vi "Stepper FPGA Solution.vi"() -> ()   [LabVIEW 2012]
uses:
  <vilib>/rvi/eio/common/nirviEmuTemplateMethod_errors.vi
  <vilib>/eio/EIONode/EIONode.xnode
panel:
  in  "Step Period":i16
  in  "Direction":bool
  in  "Enable/Disable":bool
  out "Step Period":i16
  in  "Stop":bool
  out "Edge Count":i32
  out "Heartbeat":bool
  out "Absolute Position":i16
  # "Motor Feedback"
  # "Motor Command"
  # "Calibrate Steps to Deg"
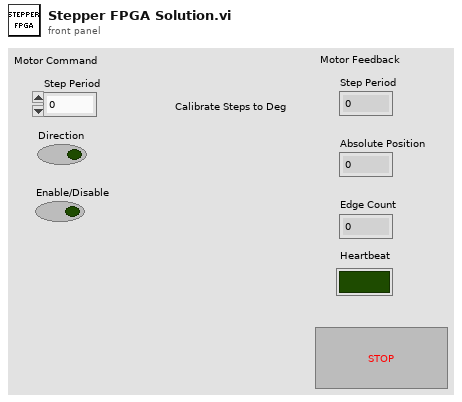
[diagram p1: front panel]
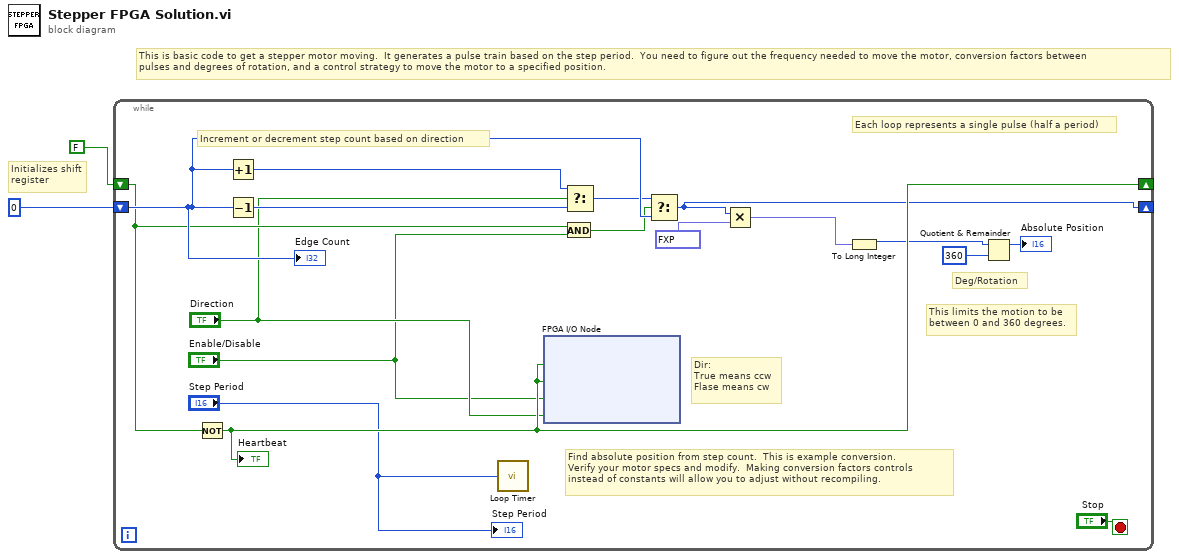
[diagram p0: block diagram]
diagram:
  # "Initializes shift\nregister"
  # "This is basic code to get a stepper motor moving.  It generates a pulse train based on the step period.  You need to figure out the frequency needed to move the motor, conversion factors between \npulses and degrees of rotation, and a control strategy to move the motor to a specified position."
  n1 = while {
    shift-right: [w9] -> _
    shift-left: i16 0 -> [w19]
    shift-right: [w16] -> _
    shift-left: FALSE -> [w17]
    stop <- "Stop" stop-if-true
    # "This limits the motion to be\nbetween 0 and 360 degrees."
    # "Deg/Rotation"
    # "Each loop represents a single pulse (half a period)"
    # "Dir:\nTrue means ccw\nFlase means cw"
    # "Find absolute position from step count.  This is example conversion.  \nVerify your motor specs and modify.  Making conversion factors controls\ninstead of constants will allow you to adjust without recompiling."
    # "Increment or decrement step count based on direction"
    n2 = Not(x=w17) -> (.not. x?=w16:bool)
    "Heartbeat" <- w16
    n3 = Increment(x=w19) -> (x+1=w15:i16)
    n4 = Decrement(x=w19) -> (x-1=w14:i16)
    n5 = call "Loop Timer"("Count(Ticks)"="Step Period") -> ()  [unwired: 1 out]
    n6 = xnode "FPGA I/O Node"("Stepper_Step"=w16, "Heartbeat LED"=w16, "Stepper_Enable"="Enable/Disable", "Stepper_Direction"="Direction") -> ()  [unwired: 4 in, 4 out]
    n7 = And(x=w17, y="Enable/Disable") -> (x .and. y?=w11:bool)
    n8 = Select(t=w15, s="Direction", f=w14) -> (s? t:f=w13:i16)
    n9 = Select(t=w13, s=w11, f=w19) -> (s? t:f=w9:i16)
    n10 = Multiply(x=w9, y=fxp<+,5,0> 0.90625) -> (x*y=w4:fxp<+/-,21,16>)
    n11 = To Long Integer(number=w4) -> (32bit integer=w3:i32)
    n12 = Quotient & Remainder(x=w3, y=i16 360) -> (x-y*floor(x/y)=→"Absolute Position":i32)  [unwired: 1 out]
    "Edge Count" <- w19
    "Step Period" <- "Step Period"
  }
